vi "Parser Cluster Configuration.vi"(8 "error in (no error)":errorcluster, 10 "Cluster in":variant, 11 "Register Name in":string) -> (0 "error out":errorcluster, 2 "Cluster Configuration":T1)   [LabVIEW 2018, in "Scalar IO Operations.lvlib"]
uses:
  Scalar IO Operations.lvlib
  TypeDefs/Cluster Configuration.ctl
  <vilib>/Utility/Data Type/Type Definitions/Data Type.ctl
  TypeDefs/Cluster Configuration Store.ctl
  TypeDefs/FXP Configuration.ctl
  <vilib>/fxp/LVFixedPointRepBitsTypeDef.ctl
  <vilib>/fxp/LVFixedPointRepRangeTypeDef.ctl
  <vilib>/Utility/Data Type/NI_Data Type.lvlib
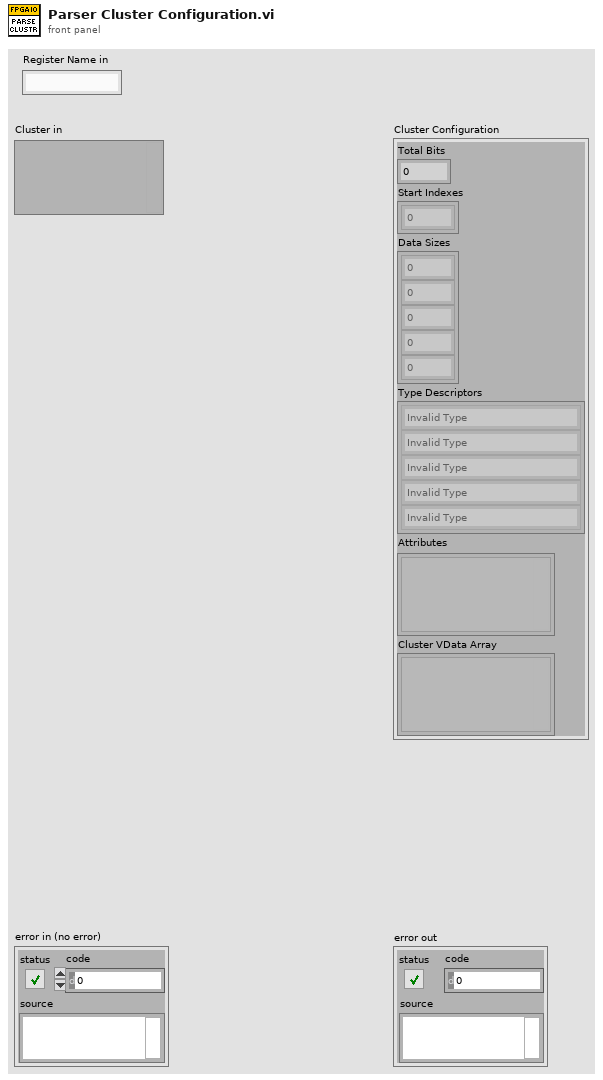
[diagram p1: front panel]
types:
  T1 = typedef "Scalar IO Operations.lvlib/Cluster Configuration.ctl" = cluster{"Total Bits":i32, "Start Indexes":i32[], "Data Sizes":i32[], "Type Descriptors":T2[], "Attributes":variant[], "Cluster VData Array":variant[]}
  T2 = typedef "NI_Data Type.lvlib/Data Type.ctl" = enum8{"Invalid Type", "Void", "I8", "I16", "I32", "I64", "U8", "U16", "U32", "U64", "Single Float", "Double Float", "Extended Float", "Single Complex", "Double Complex", "Extended Complex", "Enum U8", "Enum U16", "Enum U32", "Enum U64", "Single Float With Unit", "Double Float With Unit", "Extended Float With Unit", "Single Complex with Unit", "Double Complex with Unit", "Extended Complex with Unit", "Boolean", "String", "Path", "Picture", "Tag", "Array", "Cluster", "Variant", "LV Variant", "Waveform", "Timestamp", "Digital Waveform", "Digital Data", "ExpressData", "Refnum", "External Data", "VI", "Poly VI", "LabVIEW Class Instance", "Fixed Point"}
  T3 = typedef "Scalar IO Operations.lvlib/Cluster Configuration Store.ctl" = cluster{"Register Names":string[], "Cluster Configurations":T1[]}
  T4 = typedef "Scalar IO Operations.lvlib/FXP Configuration.ctl" = cluster{"FXP Representation":T5, "FXP Range":T6}
  T5 = typedef "LVFixedPointRepBitsTypeDef.ctl" = cluster{"Signed":bool, "Word Length":u32, "Integer Word Length":i32}
  T6 = typedef "LVFixedPointRepRangeTypeDef.ctl" = cluster{"Range Min":dbl, "Range Max":dbl, "Delta":dbl}
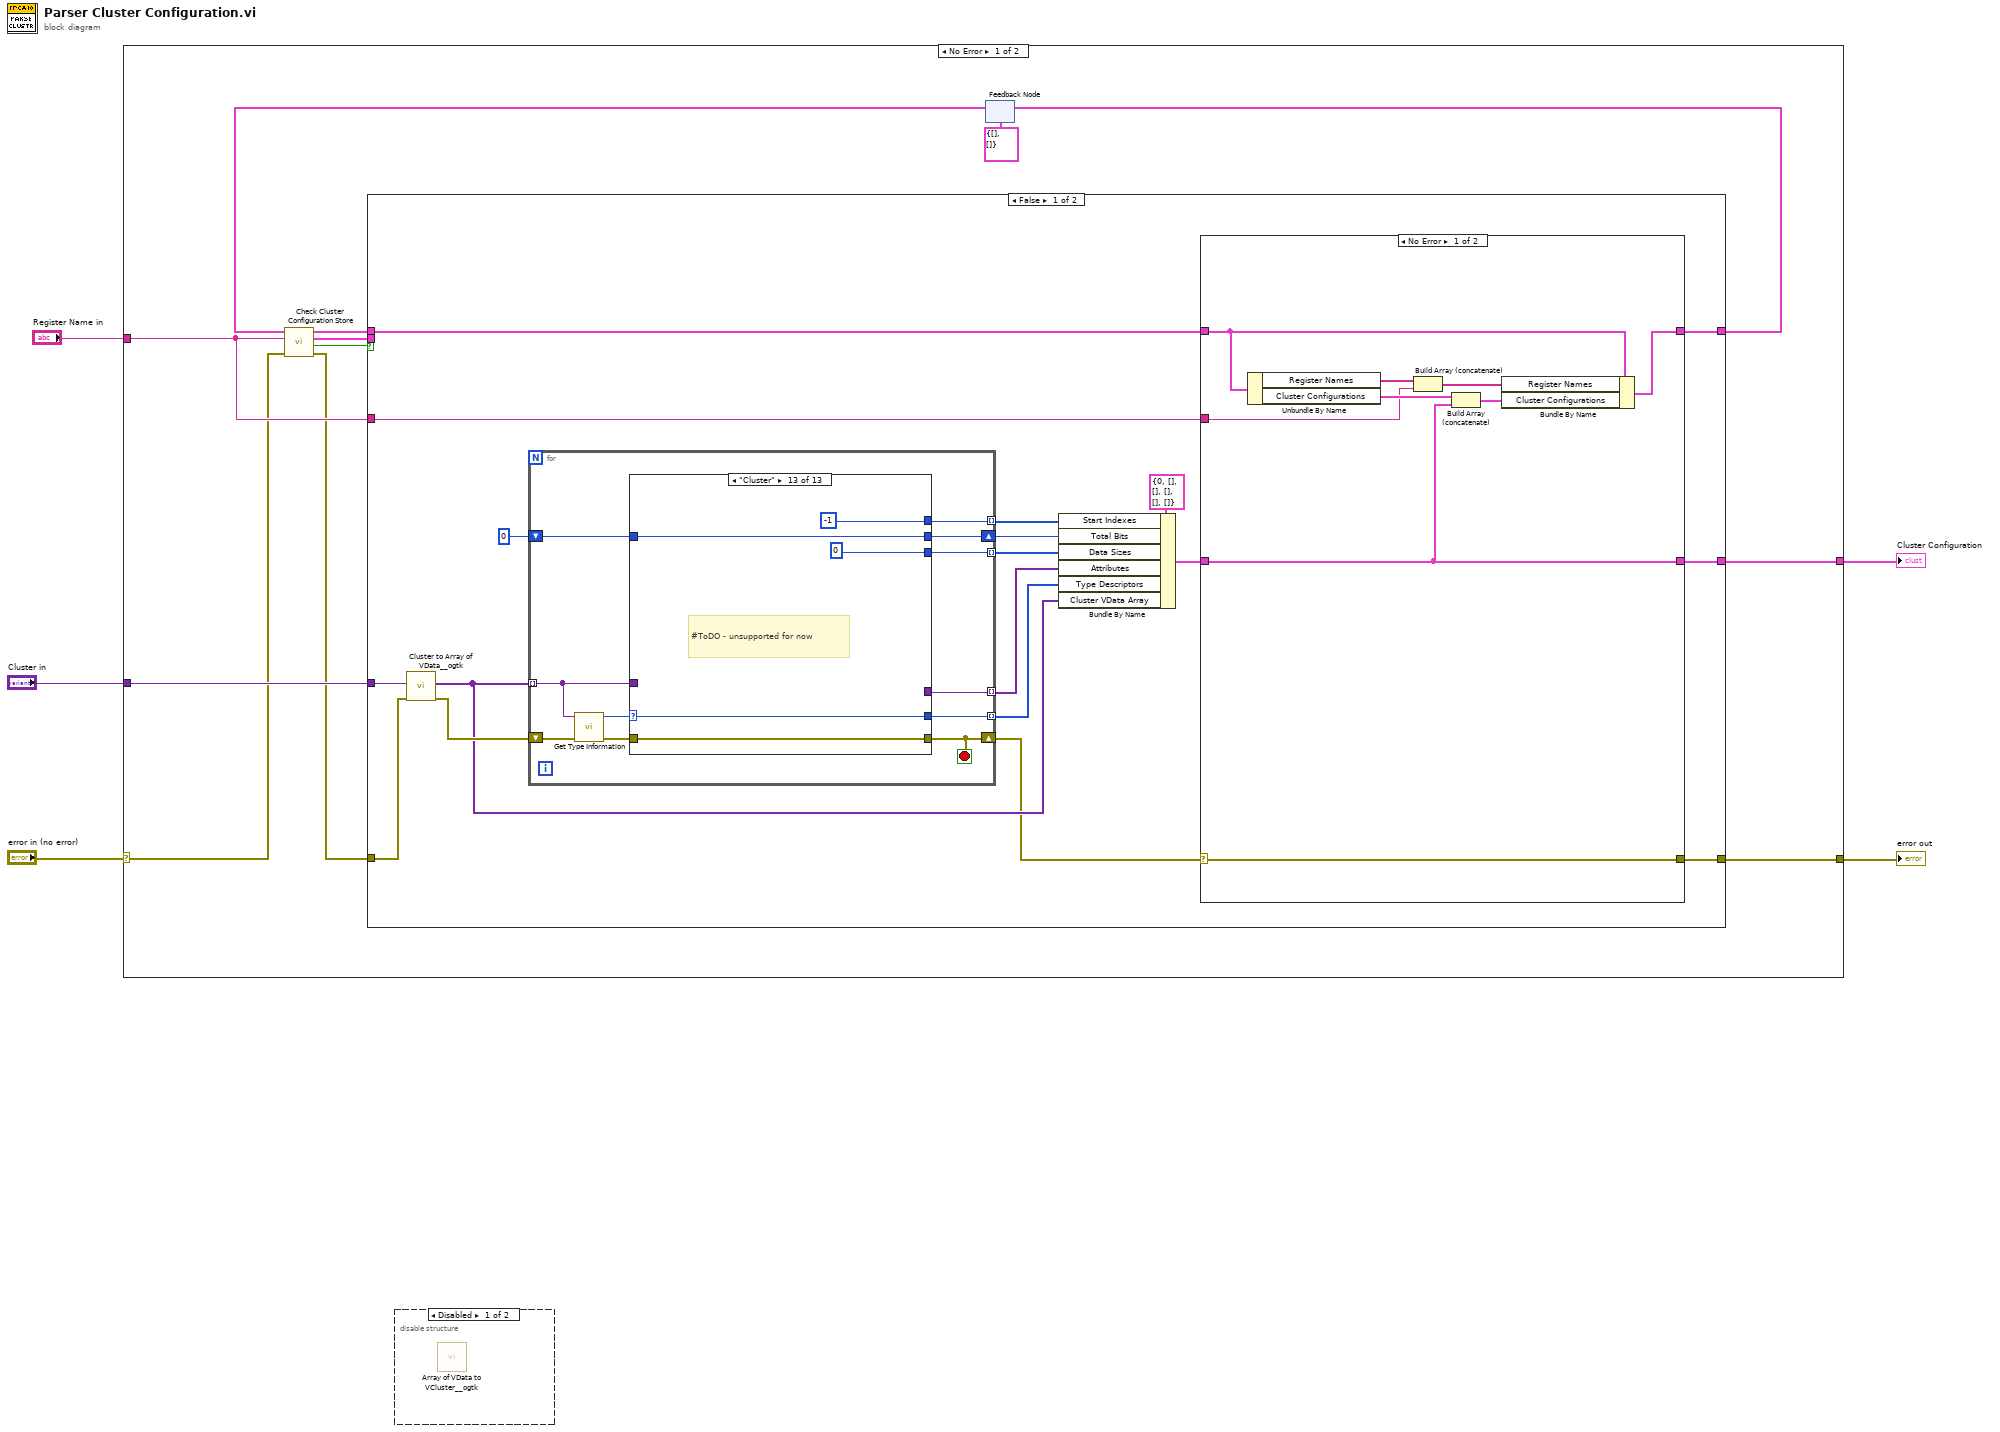
[diagram p0: block diagram]
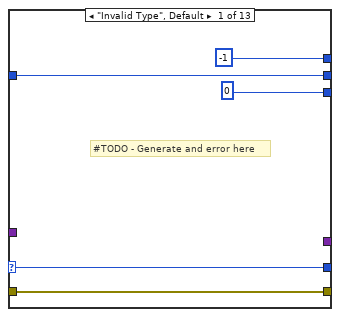
[diagram p3: hidden frame]
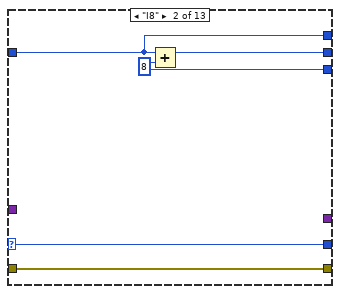
[diagram p4: hidden frame]
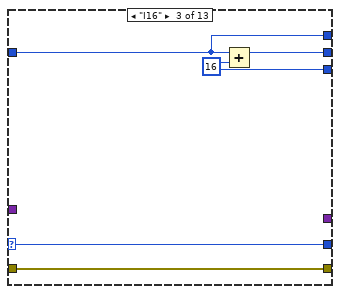
[diagram p5: hidden frame]
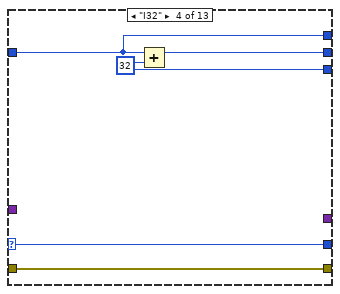
[diagram p6: hidden frame]
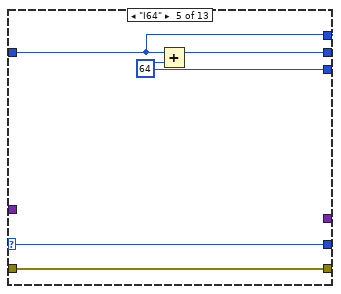
[diagram p7: hidden frame]
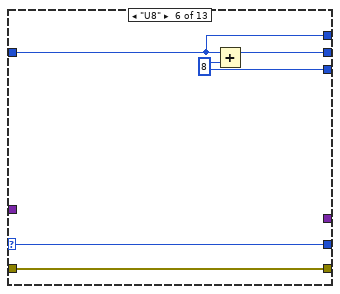
[diagram p8: hidden frame]
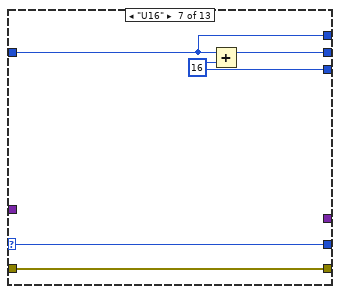
[diagram p9: hidden frame]
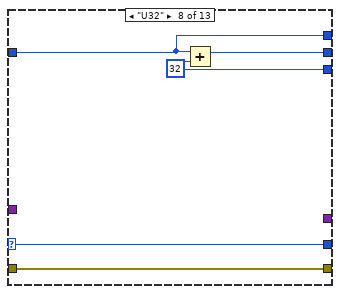
[diagram p10: hidden frame]
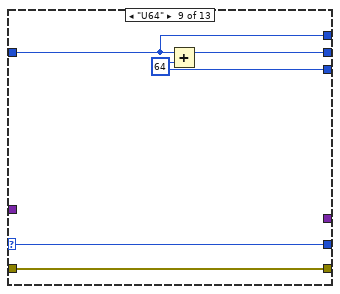
[diagram p11: hidden frame]
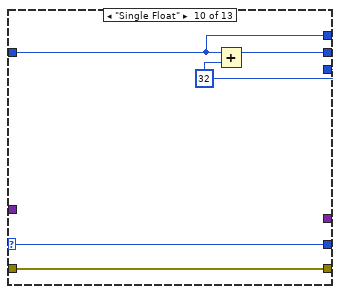
[diagram p12: hidden frame]
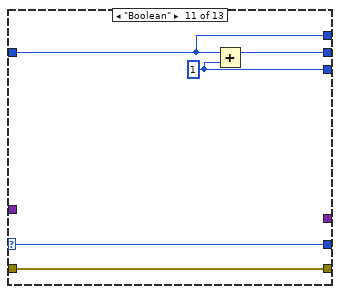
[diagram p13: hidden frame]
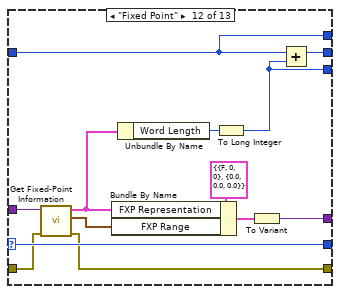
[diagram p14: hidden frame]
diagram:
  n1 = case shown="No Error" "error in (no error)" {
    selector: "error in (no error)" -> [w7 w135]
    tunnel: "Cluster in" -> [w16 _]
    tunnel: [w17 w135] -> w3
    tunnel: "Register Name in" -> [w13 _]
    tunnel: [w8 _] -> w1
    frame No Error {
      n2 = feedback #1(T3 {"Register Names"=[], "Cluster Configurations"=[]} ("Cluster Configuration Store out")) -> (w11:T3)
      n3 = call "Check Cluster Configuration Store.vi"("error in (no error)"=w7, "register name"=w13, "Cluster Configuration Store in"=w11) -> ("error IO"=w6:errorcluster, "Found"=w15:bool, "Cluster Configuration out"=w10:T1, "Cluster Configuration Store out"=w14:T3)  [unwired: 5 in]
      n4 = case shown="False" w15 {
        tunnel: w16 -> [w26 _]
        tunnel: w6 -> [w28 w134]
        tunnel: [w23 w134] -> w17
        tunnel: w14 -> [w21 w133]
        tunnel: w13 -> [w20 _]
        tunnel: [w19 w133] -> w12
        tunnel: w10 -> [_ w132]
        tunnel: [w18 w132] -> w8
        frame False {
          n5 = call <userlib>:"Cluster to Array of VData__ogtk.vi"("error in (no error)"=w28, "Cluster"=w26) -> ("error out"=w27:errorcluster, "Array of VData"=w25:variant[])  [unwired: 8 in]
          n6 = for {
            tunnel: w25 -> [w57] mode=indexing
            shift-right: [w55] -> w33
            shift-left: 0 -> [w56]
            tunnel: [w54] -> w29 mode=indexing
            tunnel: [w53] -> w30 mode=indexing
            tunnel: [w52] -> w32 mode=indexing
            tunnel: [w51] -> w31 mode=indexing
            shift-right: [w48] -> w24
            shift-left: w27 -> [w50]
            stop <- w48 stop-if-true
            n7 = call <vilib>:"Get Type Information.vi"("error in (no error)"=w50, "Variant"=w57) -> ("error out"=w49:errorcluster, "Type"=w58:T2)  [unwired: 5 in, 3 out]
            n8 = case shown="\"Cluster\"" w58 {
              selector: w58 -> [w61 w66 w71 w76 w81 w86 w91 w96 w101 w106 w111 w122 w130]
              tunnel: w57 -> [_ _ _ _ _ _ _ _ _ _ _ w126 _]
              tunnel: w56 -> [w63 w67 w72 w77 w82 w87 w92 w97 w102 w107 w112 w123 w131]
              tunnel: [w63 w68 w73 w78 w83 w88 w93 w98 w103 w108 w113 w124 w131] -> w55
              tunnel: [-1 w67 w72 w77 w82 w87 w92 w97 w102 w107 w112 w123 -1] -> w54
              tunnel: [w61 w66 w71 w76 w81 w86 w91 w96 w101 w106 w111 w122 w130] -> w53
              tunnel: [0 ("y") w65 w70 w75 w79 w85 w90 w95 w100 w105 w110 w121 0 ("y")] -> w52
              tunnel: [_ _ _ _ _ _ _ _ _ _ _ w116 _] -> w51
              tunnel: w49 -> [w59 w64 w69 w74 w80 w84 w89 w94 w99 w104 w109 w115 w127]
              tunnel: [w59 w64 w69 w74 w80 w84 w89 w94 w99 w104 w109 w114 w127] -> w48
              frame "Invalid Type", Default {
                # "#TODO - Generate and error here"
              }
              frame "I8" {
                w65 = 8 ("y")
                n9 = Add(x=w67, y=w65) -> (x+y=w68:i32)
              }
              frame "I16" {
                w70 = 16 ("y")
                n10 = Add(x=w72, y=w70) -> (x+y=w73:i32)
              }
              frame "I32" {
                w75 = 32 ("y")
                n11 = Add(x=w77, y=w75) -> (x+y=w78:i32)
              }
              frame "I64" {
                w79 = 64 ("y")
                n12 = Add(x=w82, y=w79) -> (x+y=w83:i32)
              }
              frame "U8" {
                w85 = 8 ("y")
                n13 = Add(x=w87, y=w85) -> (x+y=w88:i32)
              }
              frame "U16" {
                w90 = 16 ("y")
                n14 = Add(x=w92, y=w90) -> (x+y=w93:i32)
              }
              frame "U32" {
                w95 = 32 ("y")
                n15 = Add(x=w97, y=w95) -> (x+y=w98:i32)
              }
              frame "U64" {
                w100 = 64 ("y")
                n16 = Add(x=w102, y=w100) -> (x+y=w103:i32)
              }
              frame "Single Float" {
                w105 = 32 ("y")
                n17 = Add(x=w107, y=w105) -> (x+y=w108:i32)
              }
              frame "Boolean" {
                w110 = 1 ("y")
                n18 = Add(x=w112, y=w110) -> (x+y=w113:i32)
              }
              frame "Fixed Point" {
                n19 = call <vilib>:"Get Fixed-Point Information.vi"("error in (no error)"=w115, "Variant"=w126) -> ("error out"=w114:errorcluster, "FXP Range"=w119:T6, "FXP Representation"=w118:T5)  [unwired: 6 in, 1 out]
                n20 = Bundle By Name(cluster=T4 {"FXP Representation"={"Signed"=FALSE, "Word Length"=0, "Integer Word Length"=0}, "FXP Range"={"Range Min"=0.0, "Range Max"=0.0, "Delta"=0.0}} ("FXP Configuration"), "FXP Representation"=w118, "FXP Range"=w119) -> (w117:T4)
                n21 = Unbundle By Name(w118) -> ("Word Length"=w125:u32)
                n22 = To Long Integer(number=w125) -> (32bit integer=w121:i32)
                n23 = To Variant(anything=w117) -> (Variant=w116:variant)
                n24 = Add(x=w123, y=w121) -> (x+y=w124:i32)
              }
              frame "Cluster" {
                # "#ToDO - unsupported for now"
              }
            }
          }
          n25 = Bundle By Name(cluster=T1 {"Total Bits"=0, "Start Indexes"=[], "Data Sizes"=[], "Type Descriptors"=[], "Attributes"=[], "Cluster VData Array"=[]} ("Cluster Configuration"), "Start Indexes"=w29, "Total Bits"=w33, "Data Sizes"=w32, "Attributes"=w31, "Type Descriptors"=w30, "Cluster VData Array"=w25) -> (w22:T1)
          n26 = case shown="No Error" w24 {
            selector: w24 -> [w44 w47]
            tunnel: [w44 w47] -> w23
            tunnel: w22 -> [w36 w45]
            tunnel: w21 -> [w40 w46]
            tunnel: w20 -> [w41 _]
            tunnel: [w37 w46] -> w19
            tunnel: [w36 w45] -> w18
            frame No Error {
              n27 = Unbundle By Name(w40) -> ("Register Names"=w43:string[], "Cluster Configurations"=w42:T1[])
              n28 = Build Array (concatenate)(w43, w41) -> (w39:string[])
              n29 = Build Array (concatenate)(w42, w36) -> (w38:T1[])
              n30 = Bundle By Name(cluster=w40, "Register Names"=w39, "Cluster Configurations"=w38) -> (w37:T3)
            }
            frame Error {
            }
          }
        }
        frame True {
        }
      }
      n31 = feedback-in #1(w12) -> ()
    }
    frame Error {
    }
  }
  "Cluster Configuration" <- w1
  "error out" <- w3
  n32 = disable-structure shown="Disabled" {
    frame Disabled {
      n33 = call <userlib>:"Array of VData to VCluster__ogtk.vi"() -> ()  [unwired: 10 in, 2 out]
    }
    frame Enabled {
    }
  }
